vi "6700C Wrapper.vi"(6 "Measurement Type":i32(ring)=1 items=["Voltage"=1, "Current"=0], 7 "States":T2, 8 "error in":errorcluster, 9 "Setting":T1={"Voltage Range"=10.0, "Voltage Level "=5.0, "Behavior (0: Regulatory Limit)"=0, "Limit (1.0 A)"=1.0} {"Limit (1.0 A)" format="%^.3e"; "Behavior (0: Regulatory Limit)" items=["Regulatory Limit", "Trip Limit"]; "Voltage Level" format="%^.3e"; "Voltage Range" format="%^.3e"}, 10 "Channel Name":string="1", 11 "VISA resource name":refnum<visa-resource-name>) -> (0 "error out":errorcluster, 3 "Measurement":dbl)   [LabVIEW 2021]
uses:
  Controls/PS States.ctl
  <instrlib>/Agilent N6700 Series/Agilent N6700 Series.lvlib
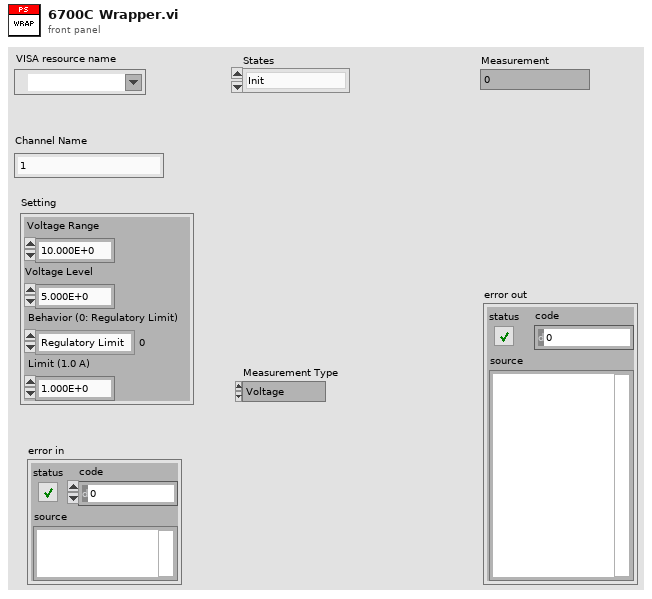
[diagram p1: front panel]
types:
  T1 = cluster{"Voltage Range":dbl, "Voltage Level ":dbl, "Behavior (0: Regulatory Limit)":i32, "Limit (1.0 A)":dbl}
  T2 = typedef "PS States.ctl" = enum16{"Init", "Config", "Enable Output", "Disable Output", "Close"}
  T3 = cluster{"Channel Name":string, "VISA resource name":refnum<visa-resource-name>}
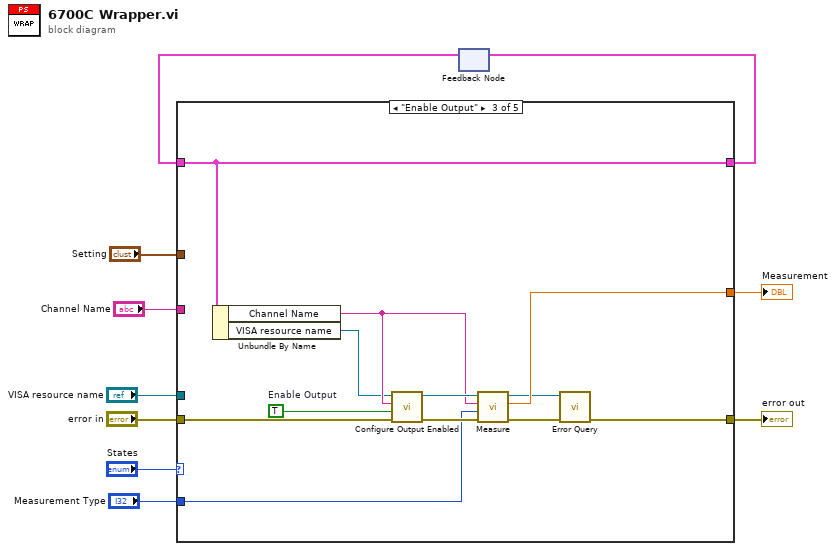
[diagram p0: block diagram]
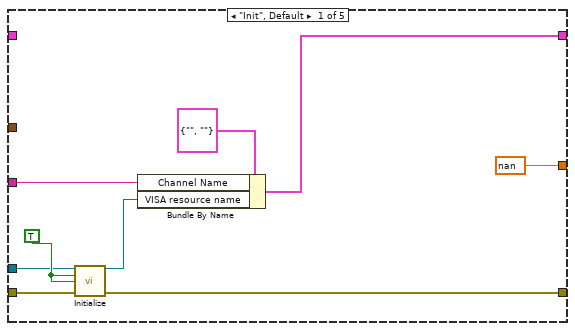
[diagram p2: hidden frame]
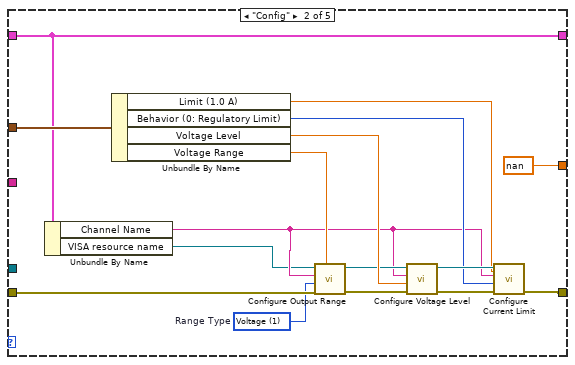
[diagram p3: hidden frame]
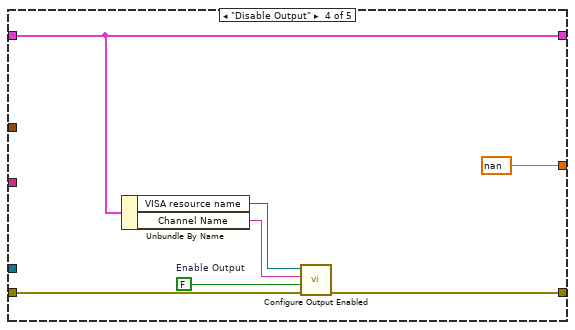
[diagram p4: hidden frame]
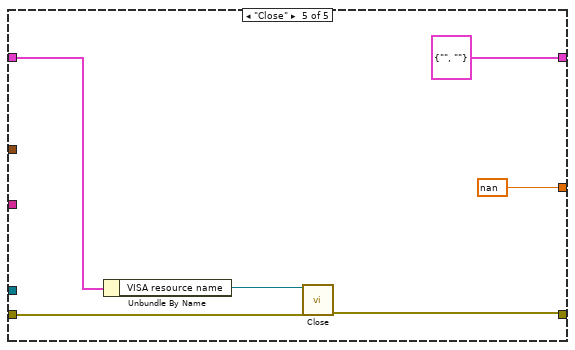
[diagram p5: hidden frame]
diagram:
  n1 = feedback #1() -> (w5:T3)  [unwired: 1 in]
  n2 = case shown="\"Enable Output\"" "States" {
    tunnel: "error in" -> [w18 w35 w45 w52 w60]
    tunnel: [w17 w27 w41 w50 w59] -> w8
    tunnel: "VISA resource name" -> [w16 _ _ _ _]
    tunnel: [w12 w23 w39 w51 T3 {"Channel Name"="", "VISA resource name"=""}] -> w6
    tunnel: w5 -> [_ w23 w39 w51 w58]
    tunnel: "Setting" -> [_ w34 _ _ _]
    tunnel: "Channel Name" -> [w14 _ _ _ _]
    tunnel: [nan nan w47 nan nan] -> w2
    tunnel: "Measurement Type" -> [_ _ w36 _ _]
    frame "Init", Default {
      w19 = TRUE ("Reset? (T: Yes)")
      n3 = call <instrlib>:"Initialize.vi"("VISA resource name"=w16, "ID Query? (T: Yes)"=w19, "Reset? (T: Yes)"=w19, "error in (no error)"=w18) -> ("VISA resource name out"=w13:refnum<visa-resource-name>, "error out"=w17:errorcluster)  [unwired: 10 in]
      n4 = Bundle By Name(cluster=T3 {"Channel Name"="", "VISA resource name"=""}, "Channel Name"=w14, "VISA resource name"=w13) -> (w12:T3)
    }
    frame "Config" {
      w26 = 1 items=["Voltage"=1, "Current"=0]  # Range Type
      n5 = Unbundle By Name(w23) -> ("Channel Name"=w22:string, "VISA resource name"=w21:refnum<visa-resource-name>)
      n6 = Unbundle By Name(w34) -> ("Limit (1.0 A)"=w28:dbl, "Behavior (0: Regulatory Limit)"=w29:i32, "Voltage Level"=w30:dbl, "Voltage Range"=w31:dbl)
      n7 = call <instrlib>:"Configure Output Range.vi"("Range (0.0)"=w31, "error in (no error)"=w35, "Range Type (1: Voltage)"=w26, "Channel Name (1)"=w22, "VISA resource name"=w21) -> ("error out"=w25:errorcluster, "VISA resource name out"=w24:refnum<visa-resource-name>)  [unwired: 5 in]
      n8 = call <instrlib>:"Configure Voltage Level.vi"("error in (no error)"=w25, "Level  (0.0 volts)"=w30, "Channel Name (1)"=w22, "VISA resource name"=w24) -> ("error out"=w33:errorcluster, "VISA resource name out"=w32:refnum<visa-resource-name>)  [unwired: 6 in]
      n9 = call <instrlib>:"Configure Current Limit.vi"("Limit (0.0 amps)"=w28, "error in (no error)"=w33, "Behavior (0: Regulatory Limit)"=w29, "Channel Name (1)"=w22, "VISA resource name"=w32) -> ("error out"=w27:errorcluster)  [unwired: 5 in, 1 out]
    }
    frame "Enable Output" {
      w46 = TRUE  # Enable Output
      n10 = Unbundle By Name(w39) -> ("Channel Name"=w38:string, "VISA resource name"=w37:refnum<visa-resource-name>)
      n11 = call <instrlib>:"Configure Output Enabled.vi"("error in (no error)"=w45, "Enable Output (False)"=w46, "Channel Name (1)"=w38, "VISA resource name"=w37) -> ("error out"=w44:errorcluster, "VISA resource name out"=w43:refnum<visa-resource-name>)  [unwired: 6 in]
      n12 = call <instrlib>:"Measure.vi"("error in (no error)"=w44, "Measurement Type (1: Voltage)"=w36, "Channel Name (1)"=w38, "VISA resource name"=w43) -> ("error out"=w42:errorcluster, "Measurement"=w47:dbl, "VISA resource name out"=w40:refnum<visa-resource-name>)  [unwired: 5 in]
      n13 = call <instrlib>:"Error Query.vi"("VISA resource name"=w40, "error in (no error)"=w42) -> ("error out"=w41:errorcluster)  [unwired: 10 in, 3 out]
    }
    frame "Disable Output" {
      w53 = FALSE  # Enable Output
      n14 = Unbundle By Name(w51) -> ("VISA resource name"=w54:refnum<visa-resource-name>, "Channel Name"=w49:string)
      n15 = call <instrlib>:"Configure Output Enabled.vi"("error in (no error)"=w52, "Enable Output (False)"=w53, "Channel Name (1)"=w49, "VISA resource name"=w54) -> ("error out"=w50:errorcluster)  [unwired: 6 in, 1 out]
    }
    frame "Close" {
      n16 = Unbundle By Name(w58) -> ("VISA resource name"=w57:refnum<visa-resource-name>)
      n17 = call <instrlib>:"Close.vi"("VISA resource name"=w57, "error in (no error)"=w60) -> ("error out"=w59:errorcluster)  [unwired: 13 in]
    }
  }
  "error out" <- w8
  "Measurement" <- w2
  n18 = feedback-in #1(w6) -> ()
